vi "LVVersionCheck_Global_OnCommand.vi"(10 "Command ID":string, 11 "Object":T1) -> ()   [LabVIEW 2015]
doc: "#translatableVI"
uses:
  <resource>/Framework/Providers/API/ItemRef.ctl
panel:
  out "error out":errorcluster
  in  "error in":errorcluster
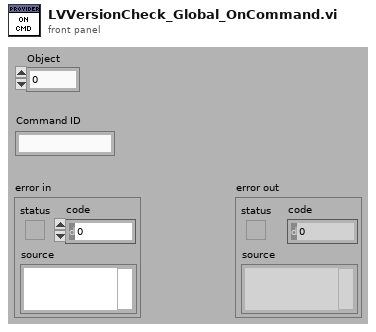
[diagram p1: front panel]
types:
  T1 = typedef "ItemRef.ctl" = u64
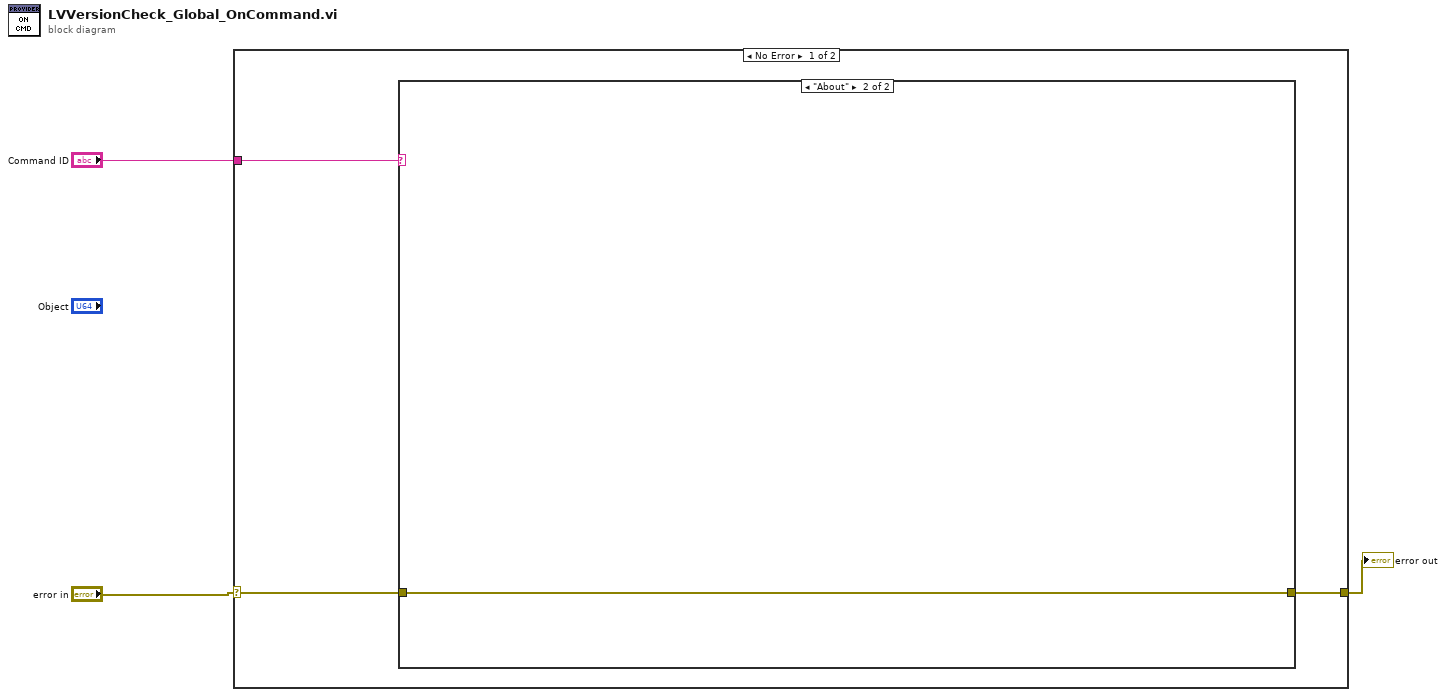
[diagram p0: block diagram]
diagram:
  n1 = case shown="No Error" "error in" {
    selector: "error in" -> [w4 w9]
    tunnel: "Command ID" -> [w6 _]
    tunnel: [w5 w9] -> w3
    frame No Error {
      n2 = case shown="\"About\"" w6 {
        tunnel: [w7 w8] -> w5
        tunnel: w4 -> [w7 w8]
        frame Default {
        }
        frame "About" {
        }
      }
    }
    frame Error {
    }
  }
  "error out" <- w3
